vi "Generate Signature.vi"(8 "error in (no error)":errorcluster, 9 "Key":string, 10 "Message":string, 11 "None in":refnum<class "None.lvclass">) -> (0 "error out":errorcluster, 2 "Signature":string, 3 "None out":refnum<class "None.lvclass">)   [LabVIEW 2020, in "Crypto.lvlib" / "None.lvclass"]
uses:
  None.lvclass
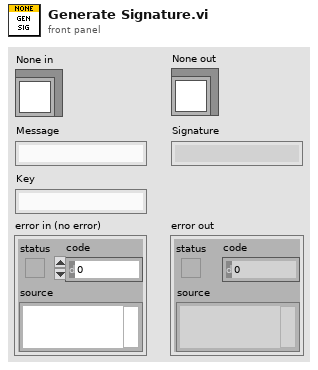
[diagram p1: front panel]
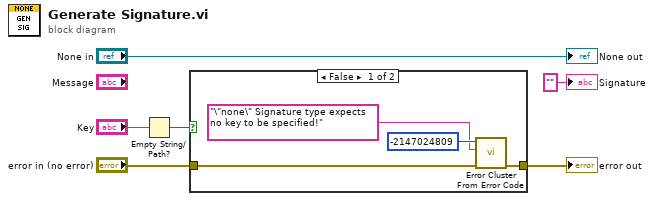
[diagram p0: block diagram]
diagram:
  n1 = Empty String/Path?(string/path="Key") -> (empty?=w4:bool)
  n2 = case shown="False" w4 {
    tunnel: "error in (no error)" -> [w7 w11]
    tunnel: [w8 w11] -> w2
    frame False {
      n3 = call <vilib>:"Error Cluster From Error Code.vi"("error in (no error)"=w7, "error message (\"\")"="\"none\" Signature type expects no key to be specified!", "error code (0)"=-2147024809) -> ("error out"=w8:errorcluster)  [unwired: 6 in]
    }
    frame True {
    }
  }
  "error out" <- w2
  "None out" <- "None in"
  "Signature" <- "" ("Signature")
